vi "alg_Determinant (SubVI).vi"(8 "에러 입력(에러 없음)":errorcluster, 11 "matrix":dbl[][](array[numeric])=[[1.0, 1.0]]) -> (0 "에러 출력":errorcluster, 2 "ans":dbl, 3 "참조 번호 출력":refnum<k35>)   [LabVIEW 2018]
uses:
  PythonConfigGlobal.vi
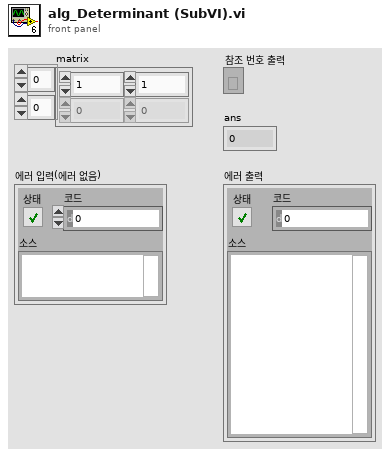
[diagram p1: front panel]
types:
  T1 = cluster{"session out":refnum<k35>, "appended path":path}
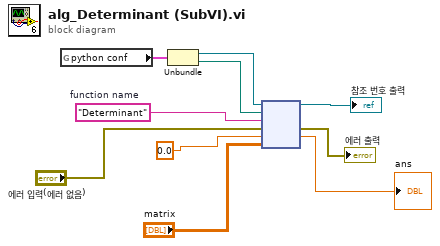
[diagram p0: block diagram]
diagram:
  w2 = "Determinant"  # function name
  n1 = global read "PythonConfigGlobal.vi" "python conf"() -> (w6:T1)
  n2 = Unbundle(w6) -> ("session out"=w4:refnum<k35>, "appended path"=w5:path)
  n3 = node(w4, w5, w2, "에러 입력(에러 없음)", 0.0 ("str1"), "matrix") -> (→"참조 번호 출력":refnum<k35>, →"에러 출력":errorcluster, →"ans":dbl)  [unwired: 1 in, 2 out]
